vi "slide.vi"() -> ()   [LabVIEW 2023]
uses:
  <vilib>/Instr/_visa.llb/VISA Configure Serial Port (Instr).vi
panel:
  in  "Tab Control":enum32{"Num Ctris", "Num Ctris i32", "Num Lnds"}(tab)
  in  "Knob":dbl(knob) scale=0.0..10.0
  in  "Dial":dbl(knob) scale=0.0..10.0
  in  "Vertical full Slide":dbl(slide) scale=0.0..10.0
  in  "Vertical Pointer Slide":dbl(slide) scale=0.0..10.0
  in  "Color Box":u32(colorbox)
  in  "Side Pointer Slide":dbl(slide) scale=0.0..10.0
  in  "Side Full Slide":dbl(slide) scale=0.0..10.0
  in  "Num Ctrl":dbl
  out "Numeric":dbl
  out "Side Full":dbl
  out "Side Pointer":dbl
  out "Vertical Full":dbl
  out "Vertical Pointer":dbl
  out "Knob_Value":dbl
  out "Dial Value":dbl
  out "Color Value":u32 format="%x"
  in  "Knob 2":i32(knob) scale=0.0..10.0
  in  "Dial 2":i32(knob) scale=0.0..10.0
  in  "Vertical full Slide 2":i32(slide) scale=0.0..10.0
  in  "Vertical Pointer Slide  2":i32(slide) scale=0.0..10.0
  in  "Color Box 2":u32(colorbox)
  in  "Side Pointer Slide  2":i32(slide) scale=0.0..10.0
  in  "Side Full Slide  2":i32(slide) scale=0.0..10.0
  in  "Num Ctrl 2":i32
  out "Numeric 2":i32
  out "Side Full 2":i32
  out "Side Pointer 2":i32
  out "Vertical Full 2":i32
  out "Vertical Pointer 2":i32
  out "Knob_Value 2":i32
  out "Dial Value 2":i32
  out "Color Value 2":u32 format="%x"
  in  "stop":bool
  out "read buffer":string
  in  "baud rate (9600)":u32=9600
  in  "VISA resource name":refnum<visa-resource-name>
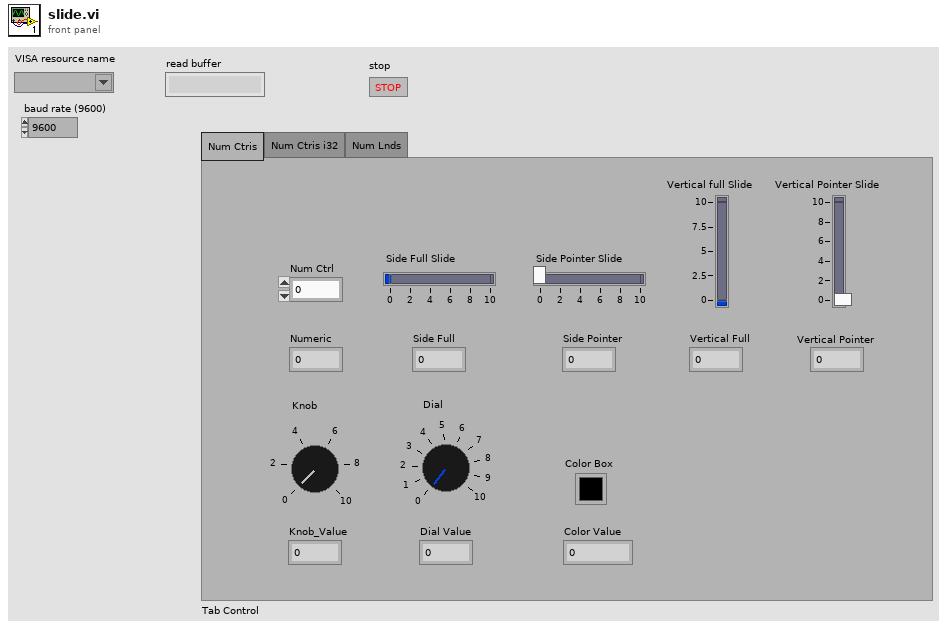
[diagram p1: front panel]
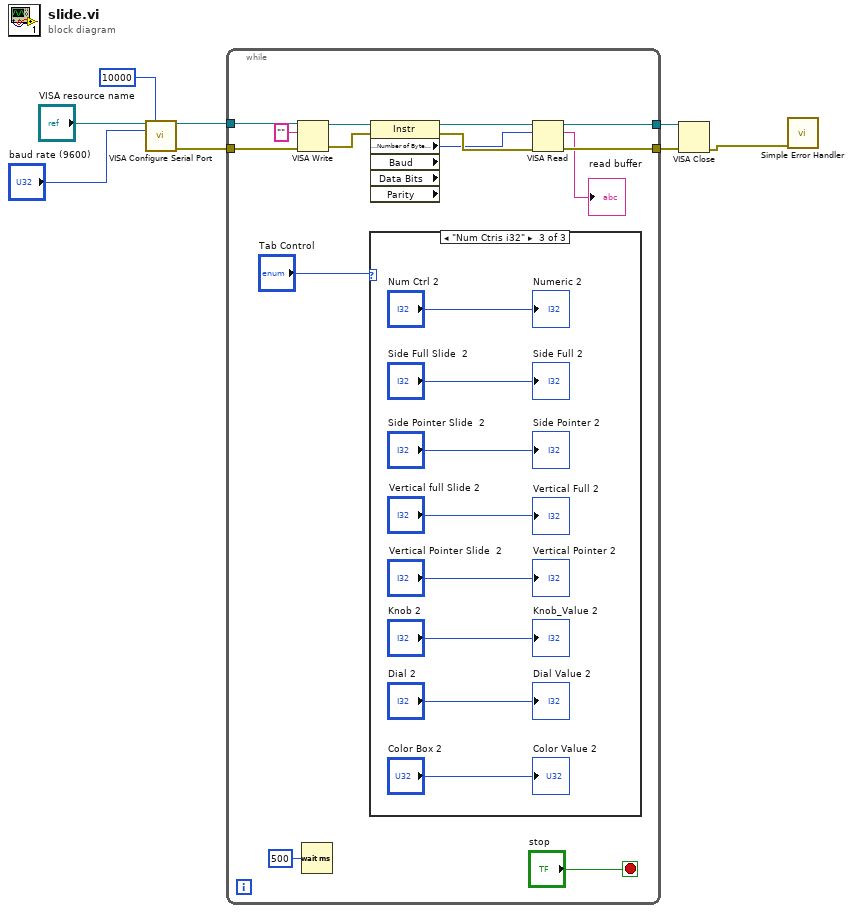
[diagram p0: block diagram]
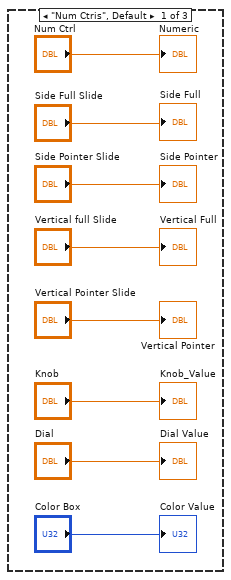
[diagram p2: hidden frame]
diagram:
  n1 = call-poly "VISA Configure Serial Port"("VISA resource name"="VISA resource name", "timeout (10sec)"=u32 10000, "baud rate (9600)"="baud rate (9600)") -> ("VISA resource name out"=w5:refnum<visa-resource-name>, "error out"=w4:errorcluster)  [unwired: 11 in]
  n2 = while {
    tunnel: w5 -> [w22]
    tunnel: w4 -> [w21]
    tunnel: [w14] -> w3
    tunnel: [w13] -> w2
    stop <- "stop" stop-if-true
    n3 = VISA Write(VISA resource name=w22, write buffer="", error in (no error)=w21) -> (VISA resource name out=w20:refnum<visa-resource-name>, error out=w19:errorcluster)  [unwired: 1 out]
    n4 = Wait (ms)(milliseconds to wait=u32 500) -> ()  [unwired: 1 out]
    n5 = case shown="\"Num Ctris i32\"" "Tab Control" {
      frame "Num Ctris", Default {
        "Vertical Pointer" <- "Vertical Pointer Slide"
        "Vertical Full" <- "Vertical full Slide"
        "Side Full" <- "Side Full Slide"
        "Side Pointer" <- "Side Pointer Slide"
        "Numeric" <- "Num Ctrl"
        "Knob_Value" <- "Knob"
        "Color Value" <- "Color Box"
        "Dial Value" <- "Dial"
      }
      frame "Num Lnds" {
      }
      frame "Num Ctris i32" {
        "Color Value 2" <- "Color Box 2"
        "Side Full 2" <- "Side Full Slide  2"
        "Knob_Value 2" <- "Knob 2"
        "Numeric 2" <- "Num Ctrl 2"
        "Vertical Full 2" <- "Vertical full Slide 2"
        "Dial Value 2" <- "Dial 2"
        "Side Pointer 2" <- "Side Pointer Slide  2"
        "Vertical Pointer 2" <- "Vertical Pointer Slide  2"
      }
    }
    n6 = property class="Instr" props=["Serial Settings:Number of Bytes at Serial Port", "Baud", "Data Bits", "Parity"](reference=w20, error in=w19) -> (reference out=w18:refnum<visa-resource-name>, error out=w17:errorcluster, "Serial Settings:Number of Bytes at Serial Port"=w16:u32)  [unwired: 3 out]
    n7 = VISA Read(VISA resource name=w18, byte count=w16, error in (no error)=w17) -> (VISA resource name out=w14:refnum<visa-resource-name>, read buffer=→"read buffer":string, error out=w13:errorcluster)  [unwired: 1 out]
  }
  n8 = VISA Close(VISA resource name=w3, error in (no error)=w2) -> (error out=w1:errorcluster)
  n9 = call <vilib>:"Simple Error Handler.vi"("error in (no error)"=w1) -> ()  [unwired: 4 in, 5 out]
